vi "BeamGage Callback with notification.vi"(4 "User Parameter":T1, 6 "Control Ref":refnum<k24>, 7 "Event Common Data":T2) -> ()   [LabVIEW 2009]
doc: "A .net callback VI that queries BeamGage for Divergence measurements. Divergence results are loaded into a notifier queue than can be read by an upper level VI as new results become available."
uses:
  C:/Program Files/Spiricon/BeamGage Professional/Spiricon.BeamGage.Automation.dll
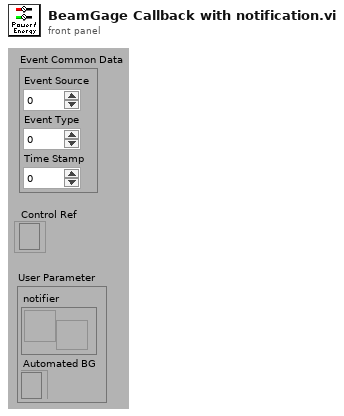
[diagram p1: front panel]
types:
  T1 = cluster{"notifier":refnum<notifier>, "Automated BG":refnum<k24>}
  T2 = cluster{"Event Source":i32, "Event Type":u32, "Time Stamp":u32}
  T3 = cluster{"Total":dbl, "Peak":dbl, "PeakLocationX":dbl, "PeakLocationY":dbl, "Width":dbl, "Height":dbl, "DoubleData":dbl[]}
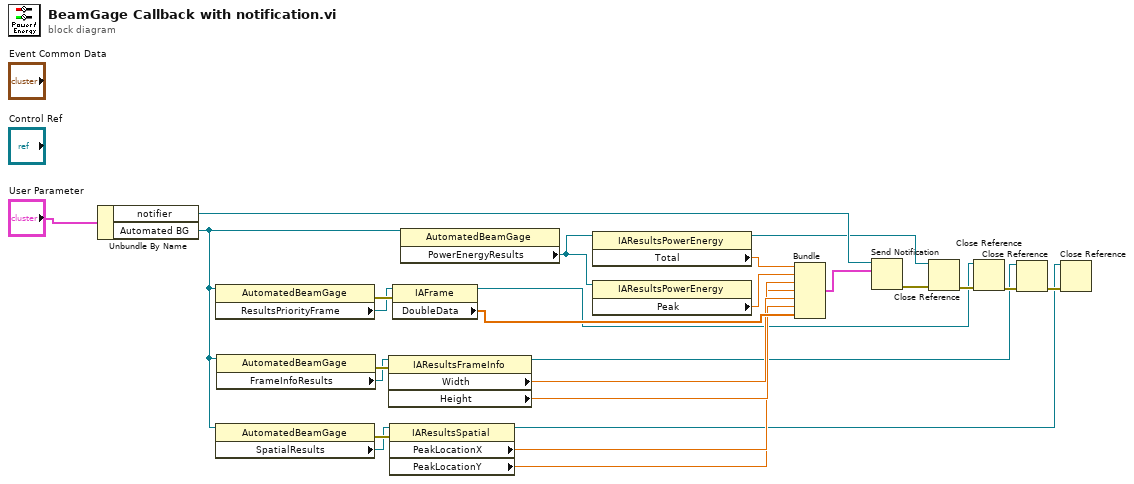
[diagram p0: block diagram]
diagram:
  n1 = Unbundle By Name("User Parameter") -> ("notifier"=w24:refnum<notifier>, "Automated BG"=w19:refnum<k24>)
  n2 = property class="AutomatedBeamGage"(reference=w19) -> (error out=w18:errorcluster, "ResultsPriorityFrame"=w6:refnum<k24>)  [unwired: 1 in, 1 out]
  n3 = property class="AutomatedBeamGage"(reference=w19) -> (error out=w13:errorcluster, "SpatialResults"=w4:refnum<k24>)  [unwired: 1 in, 1 out]
  n4 = property class="AutomatedBeamGage"(reference=w19) -> (error out=w16:errorcluster, "FrameInfoResults"=w5:refnum<k24>)  [unwired: 1 in, 1 out]
  n5 = property class="IAResultsFrameInfo"(reference=w5, error in=w16) -> (reference out=w3:refnum<k24>, "Width"=w15:dbl, "Height"=w14:dbl)  [unwired: 1 out]
  n6 = property class="IAResultsSpatial"(reference=w4, error in=w13) -> (reference out=w2:refnum<k24>, "PeakLocationX"=w12:dbl, "PeakLocationY"=w11:dbl)  [unwired: 1 out]
  n7 = property class="IAFrame"(reference=w6, error in=w18) -> (reference out=w1:refnum<k24>, "DoubleData"=w17:dbl[])  [unwired: 1 out]
  n8 = property class="AutomatedBeamGage"(reference=w19) -> ("PowerEnergyResults"=w21:refnum<k24>)  [unwired: 1 in, 2 out]
  n9 = property class="IAResultsPowerEnergy"(reference=w21) -> (reference out=w20:refnum<k24>, "Total"=w23:dbl)  [unwired: 1 in, 1 out]
  n10 = property class="IAResultsPowerEnergy"(reference=w21) -> ("Peak"=w22:dbl)  [unwired: 1 in, 2 out]
  n11 = Bundle("Total"=w23, "Peak"=w22, "PeakLocationX"=w12, "PeakLocationY"=w11, "Width"=w15, "Height"=w14, "DoubleData"=w17) -> (w10:T3)  [unwired: 1 in]
  n12 = Send Notification(notification=w10, notifier=w24) -> (error out=w26:errorcluster)  [unwired: 1 in, 1 out]
  n13 = Close Reference(reference=w20, error in (no error)=w26) -> (error out=w9:errorcluster)
  n14 = Close Reference(reference=w1, error in (no error)=w9) -> (error out=w8:errorcluster)
  n15 = Close Reference(reference=w3, error in (no error)=w8) -> (error out=w7:errorcluster)
  n16 = Close Reference(reference=w2, error in (no error)=w7) -> ()  [unwired: 1 out]
